vi "Read Analogue.vi"(8 "error in (no error)":errorcluster, 11 "Tektronix Scope in":refnum<class "Tektronix MSO5.lvclass">) -> (0 "error out":errorcluster, 2 "Waveforms":waveform(dbl)[](array[waveform]), 3 "Tektronix Scope out":refnum<class "Tektronix MSO5.lvclass">)   [LabVIEW 2025, in "Scope.lvlib" / "Tektronix MSO5.lvclass"]
uses:
  Tektronix MSO5.lvclass
  Tektronix MSO5.lvclass/Tektronix MSO5.ctl
  <instrlib>/Tektronix MSO5 Series/Drivers/Tektronix MSO5X Series.lvlib
  <instrlib>/Tektronix MSO5 Series/Drivers/Public/Data/Read (Multiple Waveforms).vi
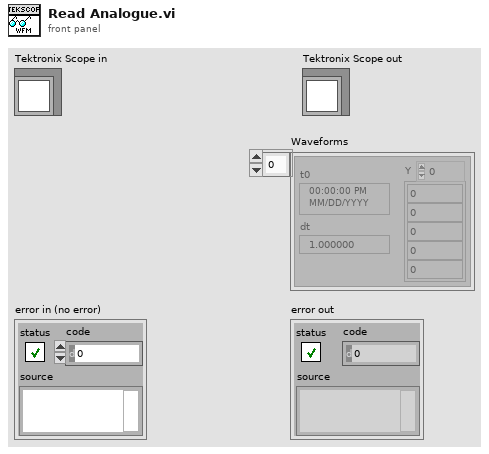
[diagram p1: front panel]
types:
  T1 = typedef "Abstract Engine.lvlibp/Abstract Instrument.lvclass/Channel.ctl" = cluster{"Alias":string, "DataType":enum16{"Anaolg Input", "Waveform"}, "Unit":enum16{"---", "V", "A", "Ohm", "Hz", "uF", "degC", "deg"}, "Upper limit":dbl, "Lower limit":dbl, "Measurement":variant}
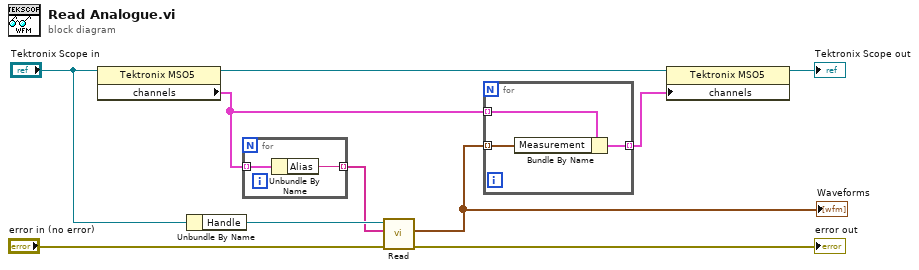
[diagram p0: block diagram]
diagram:
  n1 = property class="Tektronix MSO5"(reference="Tektronix Scope in") -> (reference out=w5:refnum<class "Tektronix MSO5.lvclass">, "channels"=w3:T1[])  [unwired: 1 in, 1 out]
  n2 = Unbundle By Name("Tektronix Scope in") -> ("Handle"=w7:refnum<visa-resource-name>)
  n3 = for {
    tunnel: w3 -> [w12] mode=indexing
    tunnel: [w11] -> w4 mode=indexing
    n4 = Unbundle By Name(w12) -> ("Alias"=w11:string)
  }
  n5 = call-poly <instrlib>:"Read.vi"("error in (no error)"="error in (no error)", "Channels"=w4, "VISA resource name"=w7) -> ("error out"=→"error out":errorcluster, "Waveform Graph"=w1:waveform(dbl)[])  [unwired: 6 in, 1 out]
  "Waveforms" <- w1
  n6 = for {
    tunnel: w1 -> [w15] mode=indexing
    tunnel: [w14] -> w2 mode=indexing
    tunnel: w3 -> [w13] mode=indexing
    n7 = Bundle By Name(cluster=w13, "Measurement"=w15) -> (w14:T1)
  }
  n8 = property class="Tektronix MSO5"(reference=w5, "channels"=w2) -> (reference out=→"Tektronix Scope out":refnum<class "Tektronix MSO5.lvclass">)  [unwired: 1 in, 1 out]
